vi "Stitching-Coordinates sorting by Y then X.vi"(9 "Y":dbl[](array[numeric])=[-12.5, -12.5, -187.5, -187.5, -187.5, -12.5, 162.5, 162.5], 11 "X":dbl[](array[numeric])=[-10.0, 11.0, -0.7, -175.7, 174.2, 174.2, 174.2, -0.8]) -> (1 "Sorted Pointers":i32[](array[numeric]), 3 "Sorted Array":dbl[][](array[numeric]))   [LabVIEW 2020]
panel:
  # "X"
  # "Y"
  # "Sorted by Y coordinate ascending order first, then by X coordinate ascending order."
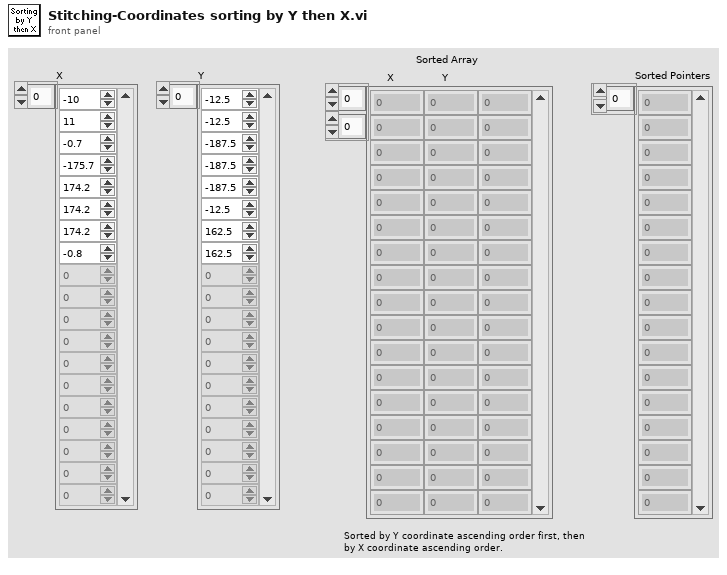
[diagram p1: front panel]
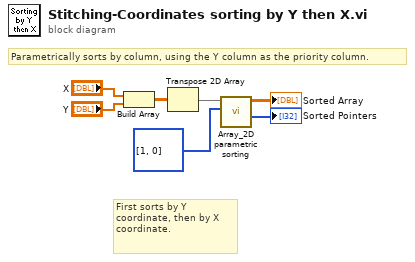
[diagram p0: block diagram]
diagram:
  # "Parametrically sorts by column, using the Y column as the priority column."
  # "First sorts by Y coordinate, then by X coordinate."
  n1 = Build Array("X", "Y") -> (w6:dbl[][])
  n2 = Transpose 2D Array(2D array=w6) -> (transposed array=w4:dbl[][])
  n3 = call "Array_2D parametric sorting.vi"("Priority Columns (1,0)"=i32[] [1, 0] ("Priority Columns"), "Unsorted Array"=w4) -> ("Sorted Pointers"=→"Sorted Pointers":i32[], "Sorted Array"=→"Sorted Array":dbl[][])  [unwired: 8 in]
